vi "MODEL SELECTION.vi"(8 "error in (no error)":errorcluster) -> (0 "error out 2":errorcluster, 2 "qr code":string[](array[string]), 3 "recipe":string)   [LabVIEW 2017]
uses:
  Global/PLC_to_Auto.vi
  <vilib>/Utility/config.llb/Read Key (String).vi
  <vilib>/Utility/config.llb/NI_LVConfig.lvlib
panel:
  in  "PART NUMBER":u16=1 min=1 max=100 step=1
  in  "PART NAME":string(combo)
  in  "CODE PREFIX":string
  in  "RECIPE SELECT":string(combo)
  in  "Cancel Button":bool
  in  "Save Button":bool
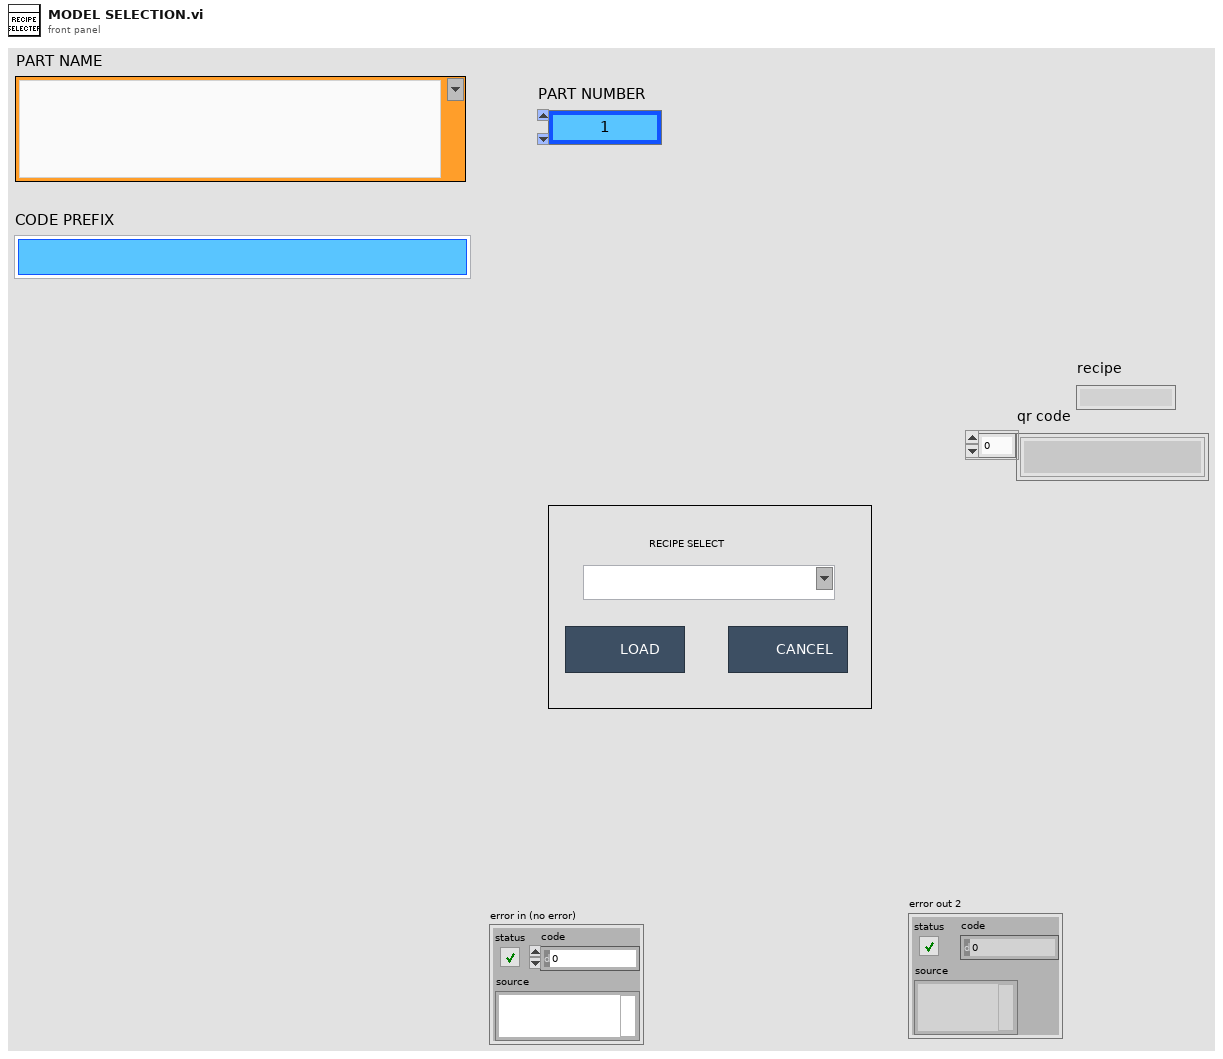
[diagram p1: front panel]
types:
  T1 = enum32{"invalid app kind", "Development System", "Run Time System", "Student Edition", "Embedded LabVIEW", "Evaluation", "Custom"}
  T2 = typedef "NI_LVConfig.lvlib/Config Data RefNum.ctl" = refnum<k1>
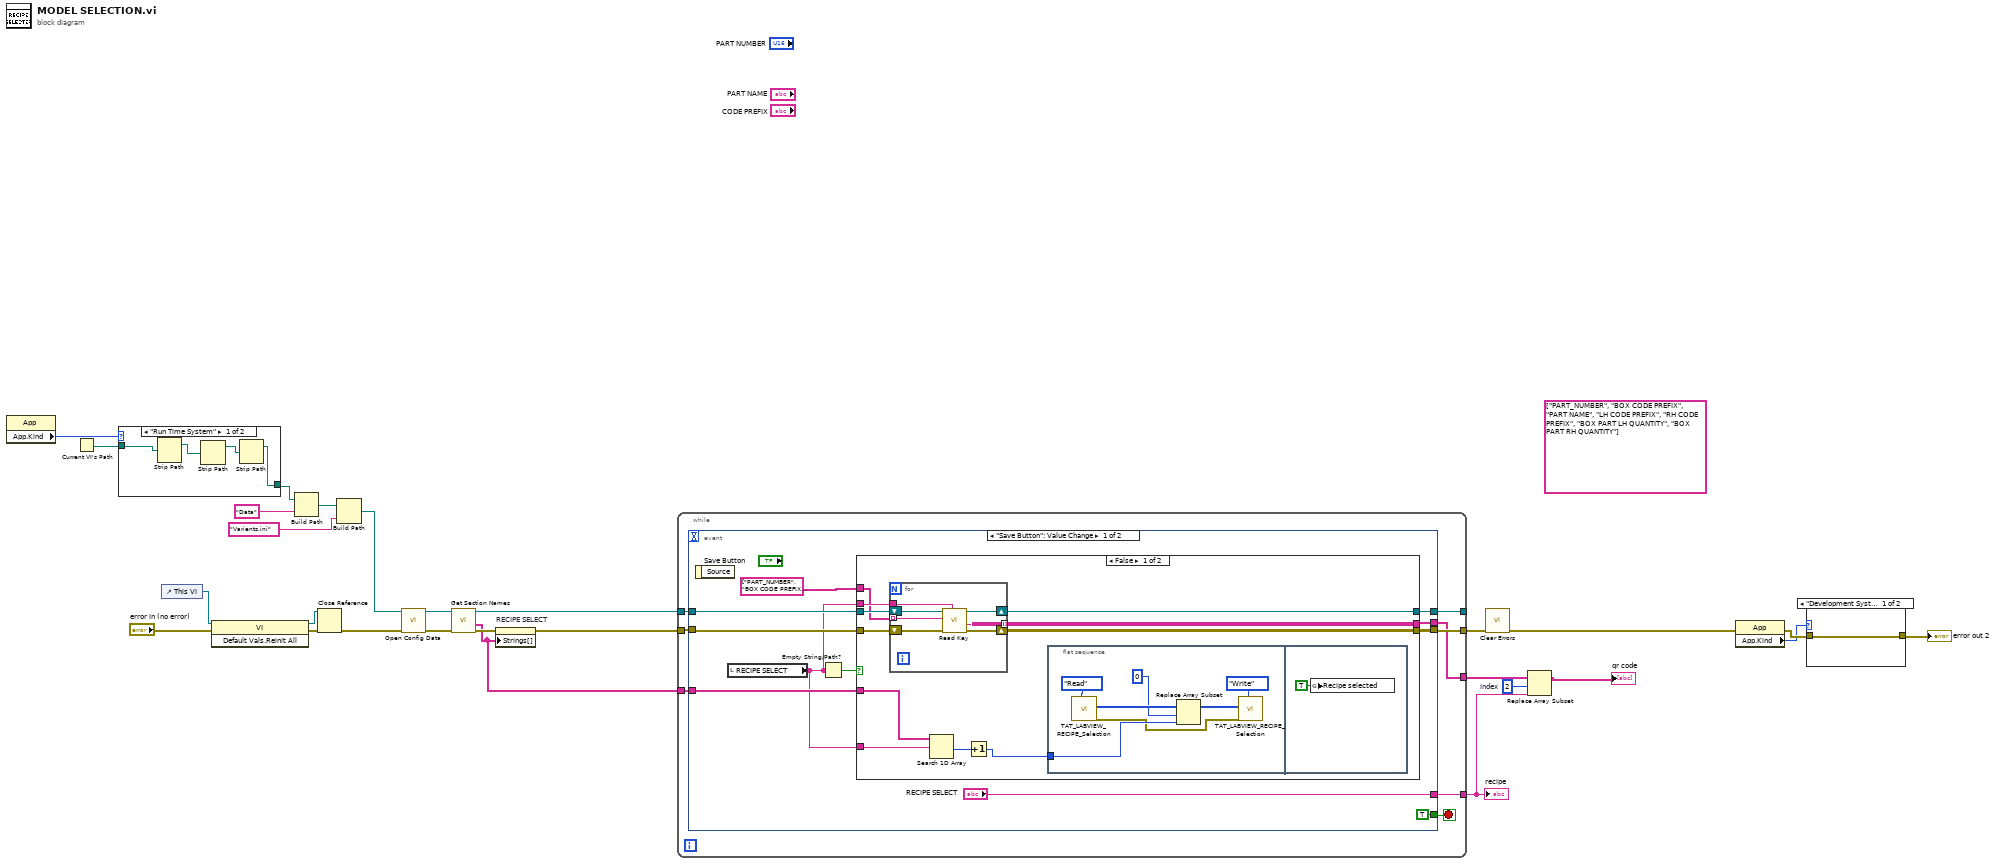
[diagram p0: block diagram]
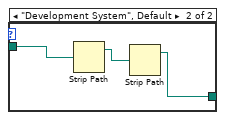
[diagram p2: hidden frame]
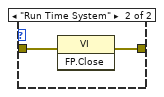
[diagram p3: hidden frame]
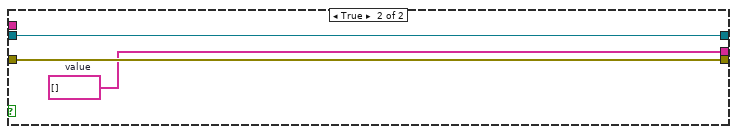
[diagram p4: hidden frame]
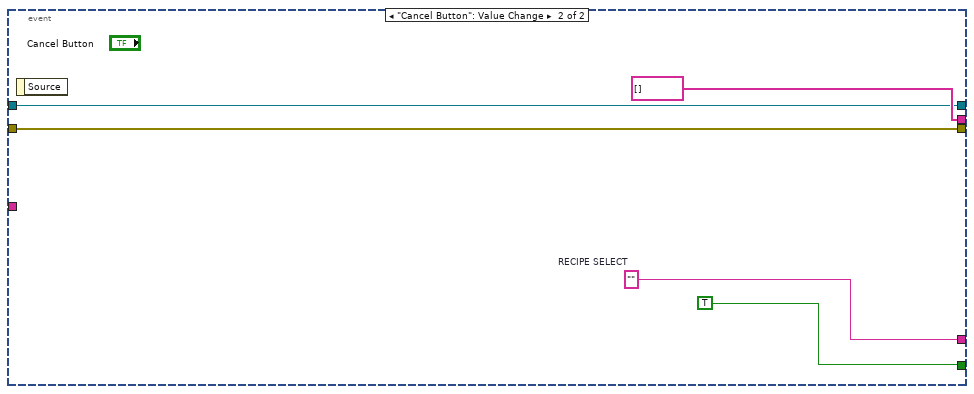
[diagram p5: hidden frame]
diagram:
  w3 = 2  # index
  (unwired) string[] ["PART_NUMBER", "BOX CODE PREFIX", "PART NAME", "LH CODE PREFIX", "RH CODE PREFIX", "BOX PART LH QUANTITY", "BOX PART RH QUANTITY"] ("Column Header Strings[]")
  n1 = property class="App"() -> ("App.Kind"=w17:T1)  [unwired: 2 in, 2 out]
  n2 = Current VI's Path() -> (path=w18:path)
  n3 = case shown="\"Run Time System\"" w17 {
    tunnel: w18 -> [w29 w33]
    tunnel: [w28 w32] -> w10
    frame "Run Time System" {
      n4 = Strip Path(path=w29) -> (stripped path=w31:path)  [unwired: 1 out]
      n5 = Strip Path(path=w31) -> (stripped path=w30:path)  [unwired: 1 out]
      n6 = Strip Path(path=w30) -> (stripped path=w28:path)  [unwired: 1 out]
    }
    frame "Development System", Default {
      n7 = Strip Path(path=w33) -> (stripped path=w34:path)  [unwired: 1 out]
      n8 = Strip Path(path=w34) -> (stripped path=w32:path)  [unwired: 1 out]
    }
  }
  n9 = control-ref of="This VI"() -> (w26:refnum<vi>)
  n10 = invoke class="VI" method="Default Vals.Reinit All"(reference=w26, error in="error in (no error)") -> (reference out=w24:refnum<vi>, error out=w23:errorcluster)  [unwired: 1 in, 1 out]
  n11 = Build Path(base path=w10, name or relative path="Data") -> (appended path=w11:path)
  n12 = Close Reference(reference=w24, error in (no error)=w23) -> (error out=w8:errorcluster)
  n13 = Build Path(base path=w11, name or relative path="Varients.ini") -> (appended path=w16:path)
  n14 = call <vilib>:"Open Config Data.vi"("error in (no error)"=w8, "configuration file path"=w16) -> ("error out"=w12:errorcluster, "refnum"=w13:T2)  [unwired: 7 in, 1 out]
  n15 = call <vilib>:"Get Section Names.vi"("error in (no error)"=w12, "refnum"=w13) -> ("error out"=w9:errorcluster, "section names"=w1:string[], "refnum out"=w6:T2)  [unwired: 7 in]
  n16 = property on="RECIPE SELECT" class="CmbBox"(error in=w9, "Strings[]"=w1) -> (error out=w7:errorcluster)  [unwired: 1 in, 1 out]
  n17 = while {
    tunnel: w7 -> [w40]
    tunnel: [w41] -> w27
    tunnel: w6 -> [w39]
    tunnel: [w38] -> _
    tunnel: [w37] -> w4
    tunnel: [w36] -> w5
    tunnel: w1 -> [w35]
    stop <- w42 stop-if-true
    n18 = event shown="[0] \"Save Button\": Value Change" {
      selector: _ -> [_ _]
      dyn-events: _ -> [_ _]
      timeout: _ -> [_ _]
      tunnel: [TRUE TRUE] -> w42
      tunnel: [w52 w86] -> w41
      tunnel: w40 -> [w51 w86]
      tunnel: w39 -> [w50 w83]
      tunnel: [w48 w83] -> w38
      tunnel: ["RECIPE SELECT" w85] -> w37
      tunnel: [w46 string[] []] -> w36
      tunnel: w35 -> [w44 _]
      event "Save Button": Value Change {
        n19 = event-data() -> ()  [unwired: 1 in, 1 out]
        n20 = local read "RECIPE SELECT"() -> (w43:string)
        n21 = Empty String/Path?(string/path=w43) -> (empty?=w49:bool)
        n22 = case shown="False" w49 {
          tunnel: [w64 w82] -> w52
          tunnel: w51 -> [w63 w82]
          tunnel: w50 -> [w62 w81]
          tunnel: w43 -> [w61 _]
          tunnel: string[] ["PART_NUMBER", "BOX CODE PREFIX", "PART NAME", "LH CODE PREFIX", "RH CODE PREFIX", "BOX PART LH QUANTITY", "BOX PART RH QUANTITY", "BOX WEIGHT"] ("Column Header Strings[]") -> [w60 _]
          tunnel: [w59 w81] -> w48
          tunnel: [w58 w80] -> w46
          tunnel: w44 -> [w57 _]
          tunnel: w43 -> [w56 _]
          frame False {
            n23 = for {
              tunnel: w61 -> [w76]
              shift-right: [w79] -> w64
              shift-left: w63 -> [w78]
              shift-right: [w74] -> w59
              shift-left: w62 -> [w77]
              tunnel: w60 -> [w75] mode=indexing
              tunnel: [w73] -> w58 mode=indexing
              n24 = call-poly <vilib>:"Read Key.vi"("section"=w76, "error in (no error)"=w78, "key"=w75, "refnum"=w77) -> ("error out"=w79:errorcluster, "value"=w73:string, "refnum out"=w74:T2)  [unwired: 4 in, 1 out]
            }
            n25 = Search 1D Array(1D array=w57, element=w56) -> (index of element=w55:i32)  [unwired: 1 in]
            n26 = Increment(x=w55) -> (x+1=w54:i32)
            n27 = flat-sequence {
              tunnel: w54 -> [w66]
              frame #0 {
                n28 = call "TAT_LABVIEW_RECIPE_Selection.vi"("Enum"=enum16{"Read", "Write"}."Read") -> ("error out"=w65:errorcluster, "Out"=w69:i32[])  [unwired: 9 in]
                n29 = Replace Array Subset(array=w69, new element=w66, index=0) -> (w67:i32[])
                n30 = call "TAT_LABVIEW_RECIPE_Selection.vi"("Enum"=enum16{"Read", "Write"}."Write", "error in (no error)"=w65, "in"=w67) -> ()  [unwired: 7 in, 2 out]
              }
              frame #1 {
                n31 = global write "PLC_to_Auto.vi" "Recipe selected"(TRUE) -> ()
              }
            }
          }
          frame True {
            w80 = string[] []  # value
          }
        }
      }
      event "Cancel Button": Value Change {
        w85 = ""  # RECIPE SELECT
        n32 = event-data() -> ()  [unwired: 1 in, 1 out]
      }
    }
  }
  "recipe" <- w4
  n33 = call <vilib>:"Clear Errors.vi"("error in (no error)"=w27) -> ("error out"=w19:errorcluster)  [unwired: 5 in, 1 out]
  n34 = Replace Array Subset(array=w5, new element=w4, index=w3) -> (→"qr code":string[])
  n35 = property class="App"(error in=w19) -> (error out=w21:errorcluster, "App.Kind"=w20:T1)  [unwired: 1 in, 1 out]
  n36 = case shown="\"Development System\", Default" w20 {
    tunnel: [w88 w90] -> w22
    tunnel: w21 -> [w88 w89]
    frame "Development System", Default {
    }
    frame "Run Time System" {
      n37 = invoke class="VI" method="FP.Close"(error in=w89) -> (error out=w90:errorcluster)  [unwired: 2 in, 2 out]
    }
  }
  "error out 2" <- w22
